vi "ImagesAndCount_Algo.vi"(8 "error in (no error)":errorcluster, 10 "ImagesAndCount":cluster{"Image Array":T1[], "ImageCount":u64}, 11 "Algorithm in":refnum<class "Algorithm.lvclass">) -> (0 "error out":errorcluster, 3 "Algorithm out":refnum<class "Algorithm.lvclass">)   [LabVIEW 2019, in "Algorithm.lvclass"]
uses:
  FrameworkOverrides/Algorithm.lvclass
  <vilib>/vision/Image Controls.llb/IMAQ Image.ctl
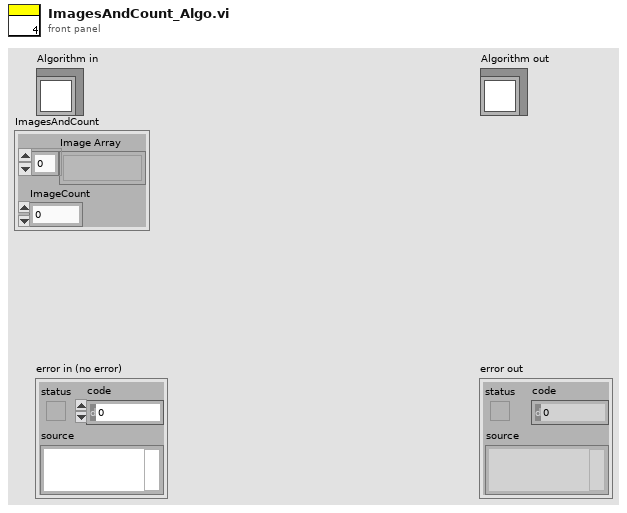
[diagram p1: front panel]
types:
  T1 = typedef "IMAQ Image.ctl" = refnum<image>
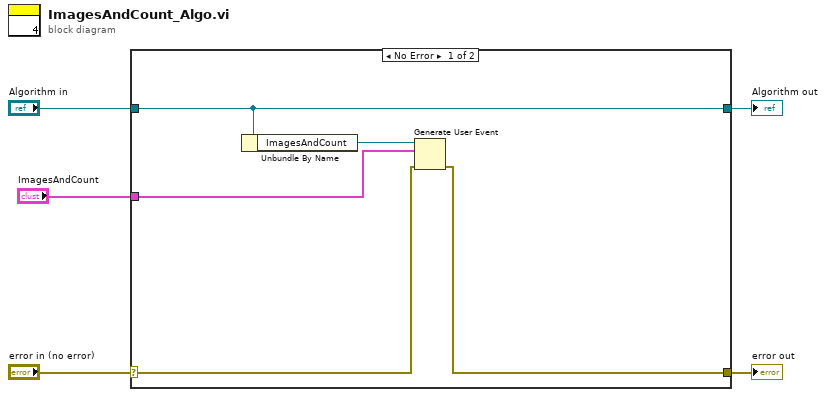
[diagram p0: block diagram]
diagram:
  n1 = case shown="No Error" "error in (no error)" {
    selector: "error in (no error)" -> [w8 w12]
    tunnel: [w7 w12] -> w4
    tunnel: [w10 w11] -> w2
    tunnel: "Algorithm in" -> [w10 w11]
    tunnel: "ImagesAndCount" -> [w6 _]
    frame No Error {
      n2 = Unbundle By Name(w10) -> ("ImagesAndCount"=w9:refnum<user-event>)
      n3 = Generate User Event(user event=w9, event data cluster=w6, error in=w8) -> (error out=w7:errorcluster)  [unwired: 1 in, 1 out]
    }
    frame Error {
    }
  }
  "error out" <- w4
  "Algorithm out" <- w2
